vi "AMI_ScanTemperature.vi"(6 "error in (no error)":errorcluster, 7 "Index":i8) -> (0 "error out":errorcluster, 1 "resulting string 2":string="                End scan temp", 2 "resulting string 1":string="                Scan Temp from 20K to 200K at 0.1K/min, in 50 steps, Uniform", 3 "Cancelled?":bool)   [LabVIEW 2017]
doc: "Use this template to create a dialog box. This template polls the state of the buttons on the front panel and does not use events. Use the Dialog Using Events template (not available in Base package) to create a dialog box with event handling."
panel:
  in  "Modo de barrido":i32(ring) items=["Solo ir", "Ir y volver"]
  in  "Approach":i32(ring) items=["FastSettle", "NoOvershoot"]
  in  "Rate (K/min)":dbl=0.1
  in  "# puntos":u32=50
  in  "Temp. Final (K)":dbl=200.0
  in  "Temp. Inicial (K)":dbl=20.0
  in  "Cancel":bool
  in  "OK":bool
  # "SCAN TEMPERATURE"
  # "Enero 2023 V2.1  a-sslcdms"
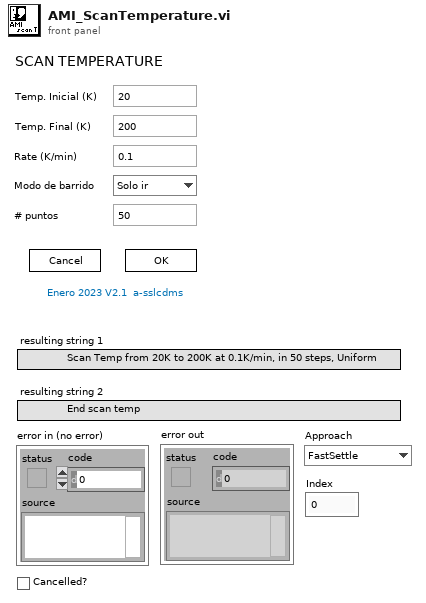
[diagram p1: front panel]
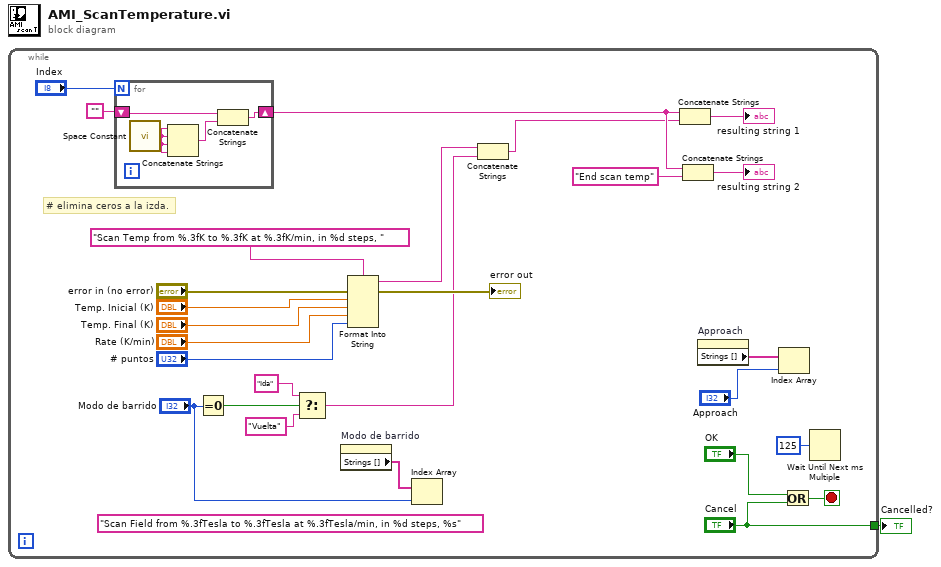
[diagram p0: block diagram]
diagram:
  n1 = while {
    tunnel: ["Cancel"] -> w1
    stop <- w27 stop-if-true
    (unwired) "Scan Field from %.3fTesla to %.3fTesla at %.3fTesla/min, in %d steps, %s" ("format string")
    # "# elimina ceros a la izda."
    n2 = for {
      N: "Index" -> [_]
      shift-right: [w31] -> w16
      shift-left: "" -> [w30]
      n3 = call <vilib>:"Space Constant.vi"() -> ("String"=w29:string)
      n4 = Concatenate Strings(w29, w29, w29, w29) -> (w32:string)
      n5 = Concatenate Strings(w30, w32) -> (w31:string)
    }
    n6 = Equal To 0?(x="Modo de barrido") -> (x = 0?=w7:bool)
    n7 = Select(t="Ida" ("resulting string 2"), s=w7, f="Vuelta" ("resulting string 2")) -> (s? t:f=w2:string)
    n8 = property on="Modo de barrido" class="Ring (strict)"() -> ("Strings []"=w3:string[])  [unwired: 2 in, 2 out]
    n9 = Format Into String(format string="Scan Temp from %.3fK to %.3fK at %.3fK/min, in %d steps, ", error in="error in (no error)", "Temp. Inicial (K)", "Temp. Final (K)", "Rate (K/min)", "# puntos") -> (resulting string=w9:string, error out=→"error out":errorcluster)  [unwired: 1 in]
    n10 = Index Array(array=w3, index="Modo de barrido") -> ()  [unwired: 1 out]
    n11 = Concatenate Strings(w9, w2) -> (w8:string)
    n12 = Concatenate Strings(w16, w8) -> (→"resulting string 1":string)
    n13 = Concatenate Strings(w16, "End scan temp" ("resulting string 2")) -> (→"resulting string 2":string)
    n14 = property on="Approach" class="Ring (strict)"() -> ("Strings []"=w14:string[])  [unwired: 2 in, 2 out]
    n15 = Index Array(array=w14, index="Approach") -> ()  [unwired: 1 out]
    n16 = Or(x="OK", y="Cancel") -> (x .or. y?=w27:bool)
    n17 = Wait Until Next ms Multiple(millisecond multiple=u32 125) -> ()  [unwired: 1 out]
  }
  "Cancelled?" <- w1
